vi "Settings_SubVI.vi"(11 "Main Data Cluster in":T1 {"task ID" format="%.0x"}) -> (3 "Main Data Cluster out":T1 {"task ID" format="%.0x"})   [LabVIEW 2024]
doc: "This SubVI updates Main Data Cluster with the info that the user provided. When \"INFO\" button is clicked github page for the project is opened.\n\nIN: Main Data Cluster in;\nOUT: Main Data Cluster out;"
uses:
  controls/#typedef_Data_Cluster.ctl
  controls/#typedef_Waveform_Type.ctl
  <vilib>/sound2/lvsound2.llb/Sound Data Format.ctl
  <vilib>/sound2/lvsound2.llb/Sound Output Task ID.ctl
  <vilib>/Platform/browser.llb/Open URL in Default Browser (string).vi
panel:
  in  "Device ID":u32
  in  "Help Button":bool
  in  "OK Button":bool
  in  "Sample Rate":dbl
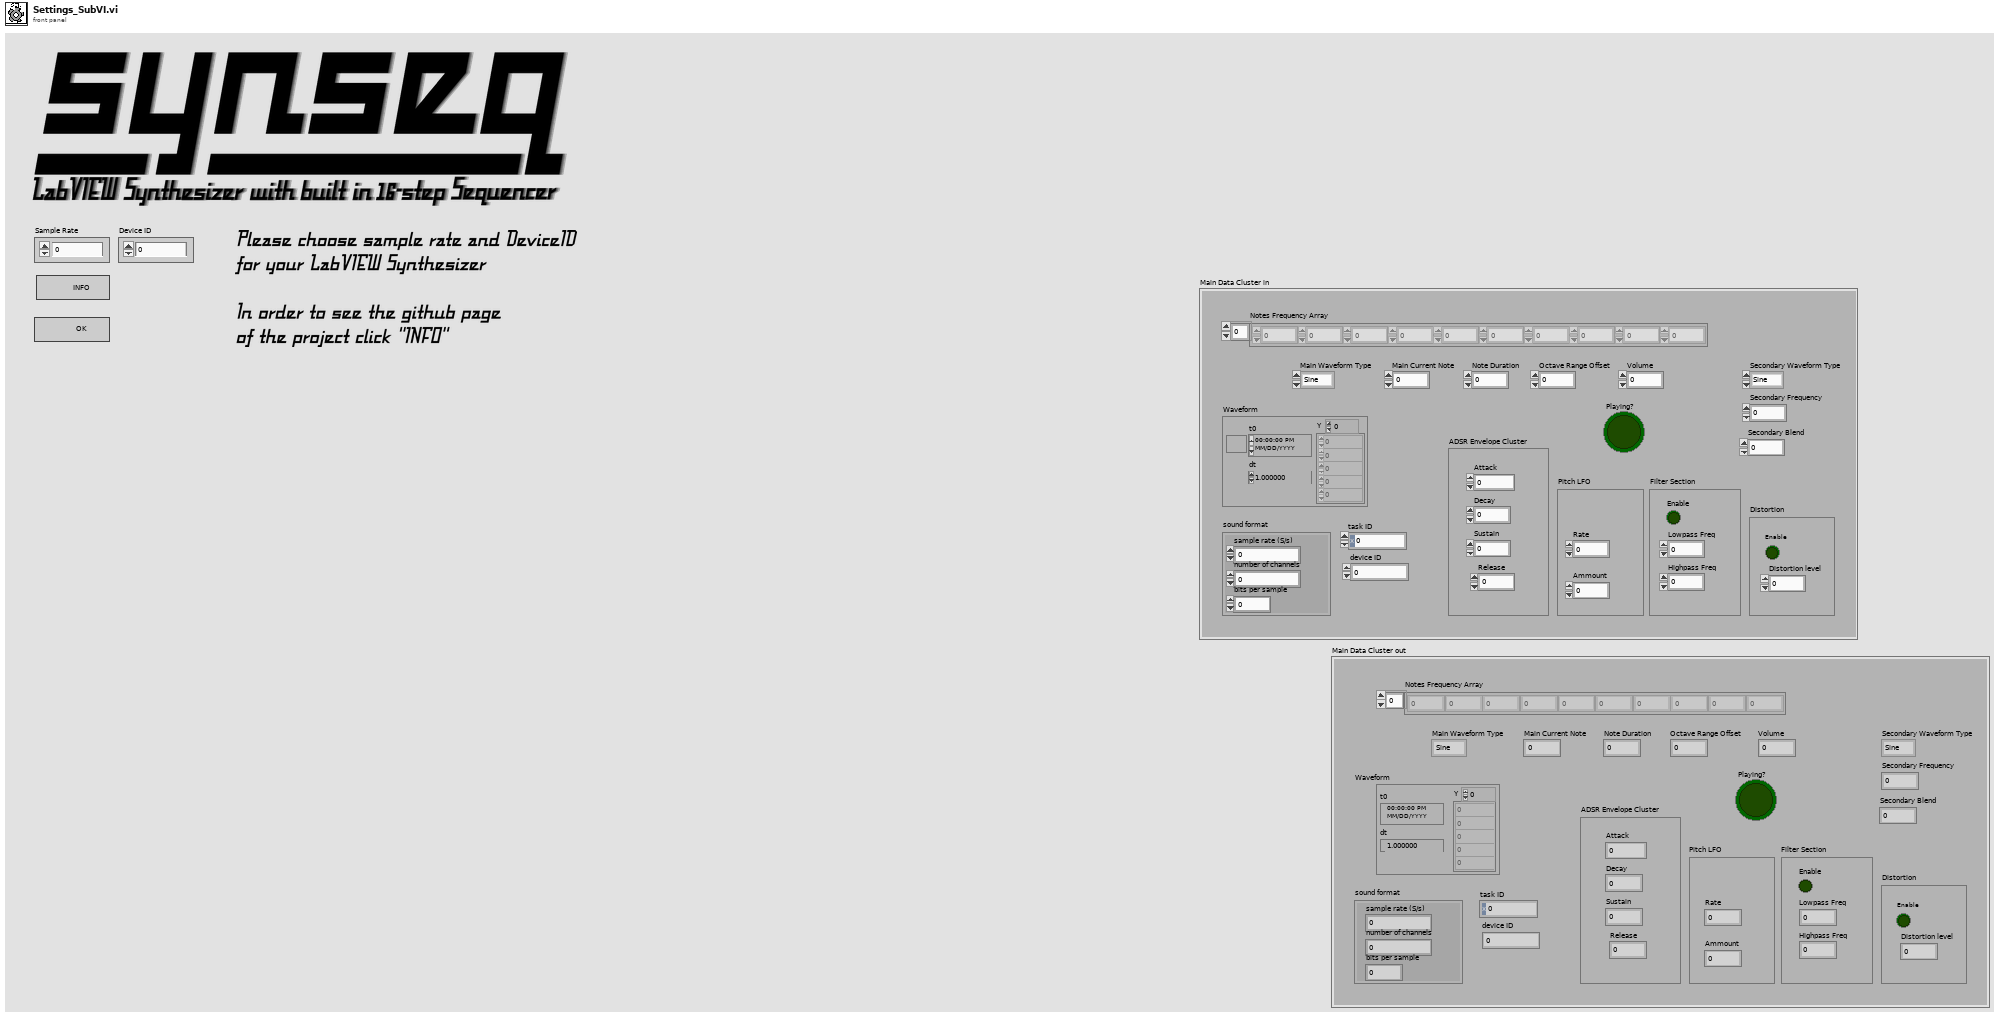
[diagram p1: front panel]
types:
  T1 = typedef "#typedef_Data_Cluster.ctl" = cluster{"Notes Frequency Array":dbl[], "Main Waveform Type":T2, "Waveform":waveform(dbl), "Main Current Note":i32, "Octave Range Offset":u32, "sound format":T3, "Task ID":T4, "Note Duration":dbl, "Volume":dbl, "ADSR Envelope Cluster":cluster{"Decay":i32, "Sustain":i32, "Attack":i32, "Release":i32}, "Playing?":bool, "Pitch LFO":cluster{"Rate":dbl, "Ammount":dbl}, "device ID":u32, "Filter Section":cluster{"Lowpass Freq":dbl, "Highpass Freq":dbl, "Enable":bool}, "Distortion":cluster{"Distortion level":dbl, "Enable":bool}, "Secondary Waveform Type":T2, "Secondary Frequency":dbl, "Secondary Blend":dbl}
  T2 = typedef "#typedef_Waveform_Type.ctl" = enum16{"Sine", "Saw", "Square", "Triangle", "Noise"}
  T3 = typedef "Sound Data Format.ctl" = cluster{"sample rate (S/s)":dbl, "number of channels":i32, "bits per sample":i32}
  T4 = typedef "Sound Output Task ID.ctl" = u32
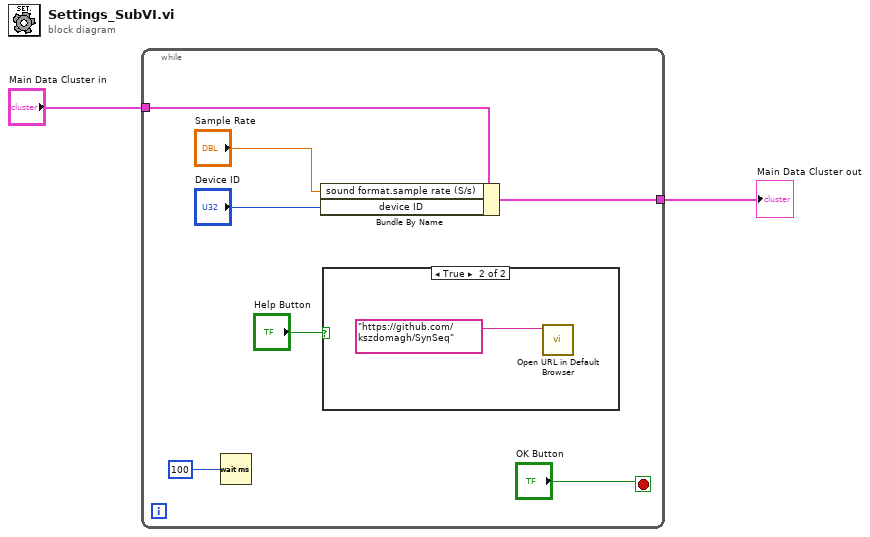
[diagram p0: block diagram]
diagram:
  n1 = while {
    tunnel: "Main Data Cluster in" -> [w9]
    tunnel: [w8] -> w1
    stop <- "OK Button" stop-if-true
    n2 = Wait (ms)(milliseconds to wait=u32 100) -> ()  [unwired: 1 out]
    n3 = Bundle By Name(cluster=w9, "sound format.sample rate (S/s)"="Sample Rate", "device ID"="Device ID") -> (w8:T1)
    n4 = case shown="True" "Help Button" {
      frame False {
      }
      frame True {
        n5 = call-poly <vilib>:"Open URL in Default Browser.vi"("URL"="https://github.com/kszdomagh/SynSeq") -> ()  [unwired: 5 in, 2 out]
      }
    }
  }
  "Main Data Cluster out" <- w1
